vi "Error Check.vi"(8 "error in (no error)":errorcluster, 10 "Modbus master in":refnum<class "Modbus Master.lvclass">, 11 "IED in":refnum<class "IED.lvclass">) -> (0 "error out":errorcluster, 2 "Modbus master out":refnum<class "Modbus Master.lvclass">, 3 "IED out":refnum<class "IED.lvclass">)   [LabVIEW 2015, in "IED Actor.lvlib" / "IED.lvclass"]
uses:
  IED.lvclass
  <vilib>/Modbus/master/Modbus Master.lvclass
  IED.lvclass/IED.ctl
  <vilib>/ActorFramework/Message Enqueuer/Message Priority.ctl
  <vilib>/ActorFramework/Actor/Actor.lvclass/Actor.ctl
  <vilib>/ActorFramework/Message Enqueuer/Message Enqueuer.lvclass/Message Enqueuer.ctl
  IED Messages/Set Modbus Handle Msg/Set Modbus Handle Msg.lvclass/Set Modbus Handle Msg.ctl
  Island Watch Actor/Island Watch Messages/Set Modbus Handle Msg/Set Modbus Handle Msg.lvclass/Set Modbus Handle Msg.ctl
  <vilib>/ActorFramework/Message Enqueuer/Init from Existing Queue.vi
  <vilib>/ActorFramework/Message Enqueuer/Enqueue.vi
  <vilib>/Modbus/master/Create Master Instance (TCP).vi
  <vilib>/ActorFramework/Message Priority Queue/Priority Enqueue.vi
  <vilib>/ActorFramework/Message Enqueuer/Message Enqueuer.lvclass
  IED Messages/Set Modbus Handle Msg/Set Modbus Handle Msg.lvclass
  Island Watch Actor/Island Watch Messages/Set Modbus Handle Msg/Set Modbus Handle Msg.lvclass
  <vilib>/ActorFramework/Stop Msg/Stop Msg.lvclass
  Utilities/Status Messaging.llb/Status Messaging.lvlib
  <vilib>/ActorFramework/Actor/Actor.lvclass
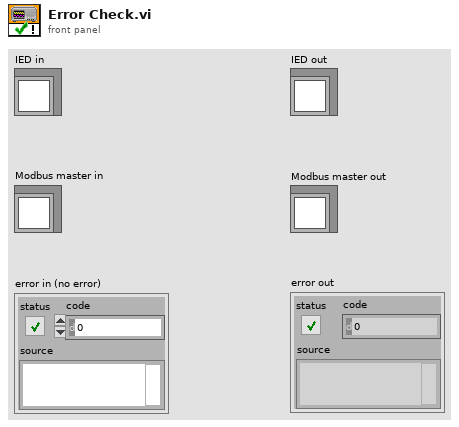
[diagram p1: front panel]
types:
  T1 = typedef "Actor Framework.lvlib/Message Enqueuer.lvclass/Message Priority.ctl" = enum16{"Low", "Normal", "High"}
  T2 = typedef "IED Actor.lvlib/IED.lvclass/Comm Cluster.ctl" = cluster{"IP Address":string, "Port":u16}
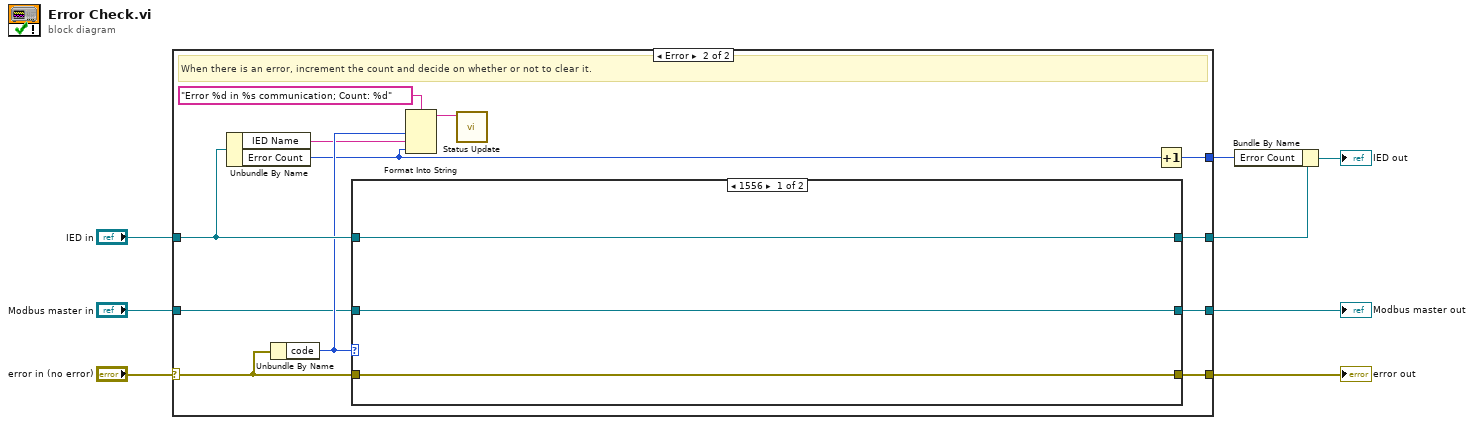
[diagram p0: block diagram]
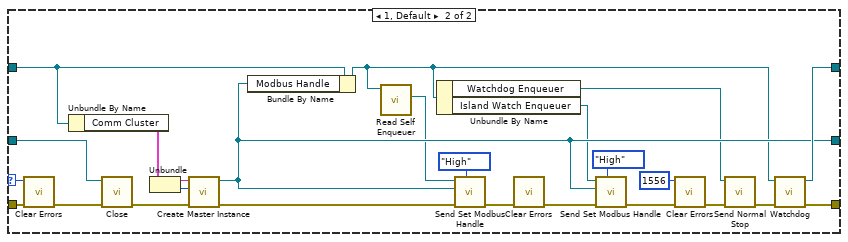
[diagram p3: hidden frame]
diagram:
  n1 = case shown="Error" "error in (no error)" {
    selector: "error in (no error)" -> [w11 w22]
    tunnel: [w11 w23] -> w8
    tunnel: "IED in" -> [w10 w19]
    tunnel: [w10 w18] -> w1
    tunnel: [_ w17] -> w4
    tunnel: "Modbus master in" -> [w9 w13]
    tunnel: [w9 w12] -> w2
    frame No Error {
      # "When there is no error, reset the count to 0."
    }
    frame Error {
      # "When there is an error, increment the count and decide on whether or not to clear it."
      n2 = Unbundle By Name(w19) -> ("IED Name"=w15:string, "Error Count"=w14:i32)
      n3 = Unbundle By Name(w22) -> ("code"=w16:i32)
      n4 = case shown="1556" w16 {
        selector: w16 -> [_ w47]
        tunnel: [w24 w51] -> w23
        tunnel: w22 -> [w24 w50]
        tunnel: w19 -> [w26 w49]
        tunnel: [w26 w48] -> w18
        tunnel: w13 -> [w25 w46]
        tunnel: [w25 w45] -> w12
        frame 1556 {
        }
        frame 1, Default {
          n5 = call <vilib>:"Clear Errors.vi"("error in (no error)"=w50, "specific error code to clear (0: all)"=w47) -> ("error out"=w44:errorcluster)  [unwired: 4 in, 1 out]
          n6 = Unbundle By Name(w49) -> ("Comm Cluster"=w39:T2)
          n7 = call-dynamic "Close.vi"("error in (no error)"=w44, "Modbus master in"=w46) -> ("error out"=w42:errorcluster)  [unwired: 9 in]
          n8 = Unbundle(w39) -> ("IP Address"=w38:string, "Port"=w37:u16)
          n9 = call-poly <vilib>:"Create Master Instance.vi"("error in (no error)"=w42, "port (502)"=w37, "address"=w38) -> ("error out"=w40:errorcluster, "TCP master instance"=w45:refnum<class "Modbus Master.lvclass">)  [unwired: 7 in]
          n10 = Bundle By Name(cluster=w49, "Modbus Handle"=w45) -> (w32:refnum<class "IED.lvclass">)
          n11 = call <vilib>:"Read Self Enqueuer.vi"("Actor"=w32) -> ("Self Enqueuer"=w41:refnum<class "Message Enqueuer.lvclass">)  [unwired: 10 in]
          n12 = Unbundle By Name(w32) -> ("Watchdog Enqueuer"=w34:refnum<class "Message Enqueuer.lvclass">, "Island Watch Enqueuer"=w30:refnum<class "Message Enqueuer.lvclass">)
          n13 = call "Send Set Modbus Handle.vi"("Message Priority (Normal)"=Message_Priority."High", "error in (no error)"=w40, "Modbus Master"=w45, "Message Enqueuer"=w41) -> ("error out"=w28:errorcluster)  [unwired: 6 in, 1 out]
          n14 = call <vilib>:"Clear Errors.vi"("error in (no error)"=w28) -> ("error out"=w27:errorcluster)  [unwired: 5 in, 1 out]
          n15 = call "Send Set Modbus Handle.vi"("Message Priority (Normal)"=Message_Priority."High", "error in (no error)"=w27, "Modbus Master"=w45, "Message Enqueuer"=w30) -> ("error out"=w31:errorcluster)  [unwired: 6 in, 1 out]
          n16 = call <vilib>:"Clear Errors.vi"("error in (no error)"=w31, "specific error code to clear (0: all)"=1556) -> ("error out"=w35:errorcluster)  [unwired: 4 in, 1 out]
          n17 = call <vilib>:"Send Normal Stop.vi"("error in (no error)"=w35, "Message Enqueuer"=w34) -> ("error out"=w33:errorcluster)  [unwired: 9 in]
          n18 = call "Watchdog.vi"("error in (no error)"=w33, "IED in"=w32) -> ("error out"=w51:errorcluster, "IED out"=w48:refnum<class "IED.lvclass">)  [unwired: 8 in]
        }
      }
      n19 = Format Into String(format string="Error %d in %s communication; Count: %d", w16, w15, w14) -> (resulting string=w20:string)  [unwired: 2 in, 1 out]
      n20 = call "Status Update.vi"("Status Update"=w20) -> ()  [unwired: 9 in, 2 out]
      n21 = Increment(x=w14) -> (x+1=w17:i32)
    }
  }
  "error out" <- w8
  "Modbus master out" <- w2
  n22 = Bundle By Name(cluster=w1, "Error Count"=w4) -> (→"IED out":refnum<class "IED.lvclass">)
